vi "General Polynomial Fit.vi"(0 "Y":dbl[](array[numeric]), 1 "polynomial order":i32=2, 2 "Coefficient Constraint":cluster{"order":i32, "coefficient":dbl}[](array[cluster]), 5 "X":dbl[](array[numeric]), 7 "Weight":dbl[](array[numeric]), 9 "tolerance":dbl=0.0001, 11 "method":T2 items=["Least Square", "Least Absolute Residual", "Bisquare"], 13 "algorithm":T1 items=["SVD", "Givens", "Givens2", "Householder", "LU Decomposition", "Cholesky", "SVD for Rank Deficient H"]) -> (4 "Best Polynomial Fit":dbl[](array[numeric]), 6 "Polynomial Coefficients":dbl[](array[numeric]), 14 "residue":dbl, 15 "error":i32)   [LabVIEW 2017, in "NI_AALPro.lvlib"]
doc: "Returns the polynomial fit of <B>polynomial order</B> for a data set (<B>X</B>, <B>Y</B>) using the Least Square, Least Absolute Residual, or Bisquare method."
uses:
  <vilib>/Analysis/NI_AALPro.lvlib
  <vilib>/Analysis/6fits.llb/Curve Fitting Criteria.ctl
  <vilib>/Analysis/6fits.llb/General Linear Fit Algorithm.ctl
panel:
  # "General Polynomial Fit"
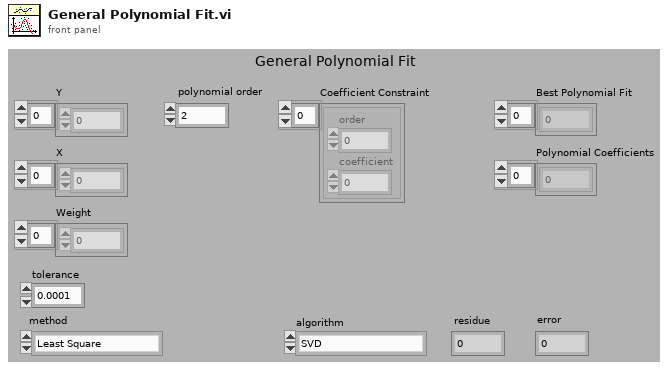
[diagram p1: front panel]
types:
  T1 = typedef "NI_AALPro.lvlib/General Linear Fit Algorithm.ctl" = u16
  T2 = typedef "NI_AALPro.lvlib/Curve Fitting Criteria.ctl" = u16
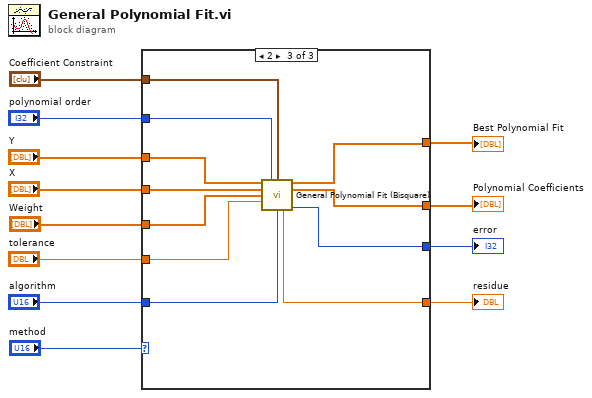
[diagram p0: block diagram]
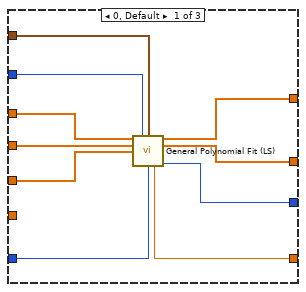
[diagram p2: hidden frame]
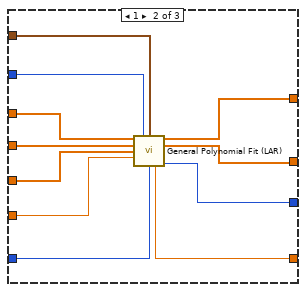
[diagram p3: hidden frame]
diagram:
  n1 = case shown="2" "method" {
    tunnel: "Coefficient Constraint" -> [w14 w24 w35]
    tunnel: "Y" -> [w22 w33 w44]
    tunnel: "X" -> [w21 w32 w43]
    tunnel: "Weight" -> [w20 w25 w42]
    tunnel: "polynomial order" -> [w13 w23 w34]
    tunnel: "algorithm" -> [w19 w30 w40]
    tunnel: [w18 w29 w39] -> w6
    tunnel: [w17 w28 w38] -> w5
    tunnel: [w16 w27 w36] -> w4
    tunnel: [w15 w26 w37] -> w3
    tunnel: "tolerance" -> [_ w31 w41]
    frame 0, Default {
      n2 = call <vilib>:"General Polynomial Fit (LS).vi"("Y"=w22, "polynomial order"=w13, "Coefficient Constraint"=w14, "X"=w21, "Weight"=w20, "algorithm"=w19) -> ("Best Polynomial Fit"=w18:dbl[], "Polynomial Coefficients"=w17:dbl[], "mse"=w16:dbl, "error"=w15:i32)  [unwired: 1 in, 5 out]
    }
    frame 1 {
      n3 = call <vilib>:"General Polynomial Fit (LAR).vi"("Y"=w33, "polynomial order"=w23, "Coefficient Constraint"=w24, "X"=w32, "Weight"=w25, "tolerance"=w31, "algorithm"=w30) -> ("Best Polynomial Fit"=w29:dbl[], "Polynomial Coefficients"=w28:dbl[], "residue"=w27:dbl, "error"=w26:i32)  [unwired: 1 in, 4 out]
    }
    frame 2 {
      n4 = call <vilib>:"General Polynomial Fit (Bisquare).vi"("Y"=w44, "polynomial order"=w34, "Coefficient Constraint"=w35, "X"=w43, "Weight"=w42, "tolerance"=w41, "algorithm"=w40) -> ("Best Polynomial Fit"=w39:dbl[], "Polynomial Coefficients"=w38:dbl[], "residue"=w36:dbl, "error"=w37:i32)  [unwired: 1 in, 4 out]
    }
  }
  "Best Polynomial Fit" <- w6
  "Polynomial Coefficients" <- w5
  "residue" <- w4
  "error" <- w3
